vi "Pulse Train demo.vi"() -> ()   [LabVIEW 2019]
doc: "This example shows how to use the Pulse Train VI to construct a series of pulses according to the user-specified pulse prototype."
uses:
  <vilib>/Analysis/1siggen.llb/General Gauss-Mod Sine.vi
  <vilib>/Analysis/1siggen.llb/General Gaussian Monopulse.vi
  <vilib>/Analysis/1siggen.llb/General Aperiodic Triangle.vi
  <vilib>/Analysis/NI_AALBase.lvlib
panel:
  in  "Amplitude & Delay":cluster{"Amplitude":dbl, "Delay (s)":dbl}[](array[cluster])=[{"Amplitude"=5.0, "Delay (s)"=1.0}, {"Amplitude"=3.0, "Delay (s)"=8.0}, {"Amplitude"=1.0, "Delay (s)"=15.0}]
  in  "Stop":bool
  in  "pulse prototype":u16(ring) items=["Gauss Mod-Sine Pattern", "Gauss Monopulse", "Triangle Pattern", "Sine Pattern"]
  in  "interpolation method":i32(ring)=1 items=["nearest", "linear", "spline", "cubic Hermite"]
  out "Pulse Prototype Graph":waveform(dbl)(graph)
  in  "delta t of pulse train":dbl=0.1
  out "Pulse Train":waveform(dbl)(graph)
  # "Overview: This example shows how to use the Pulse Train VI to construct a series of pulses.\nRequirements: LabVIEW Full Development System\nInstructions: \n1.  Run the VI.\n2. Change the pulse parameters, including the pulse prototype, and view the changes in the two graphs.  \n3. Click Stop to stop the VI."
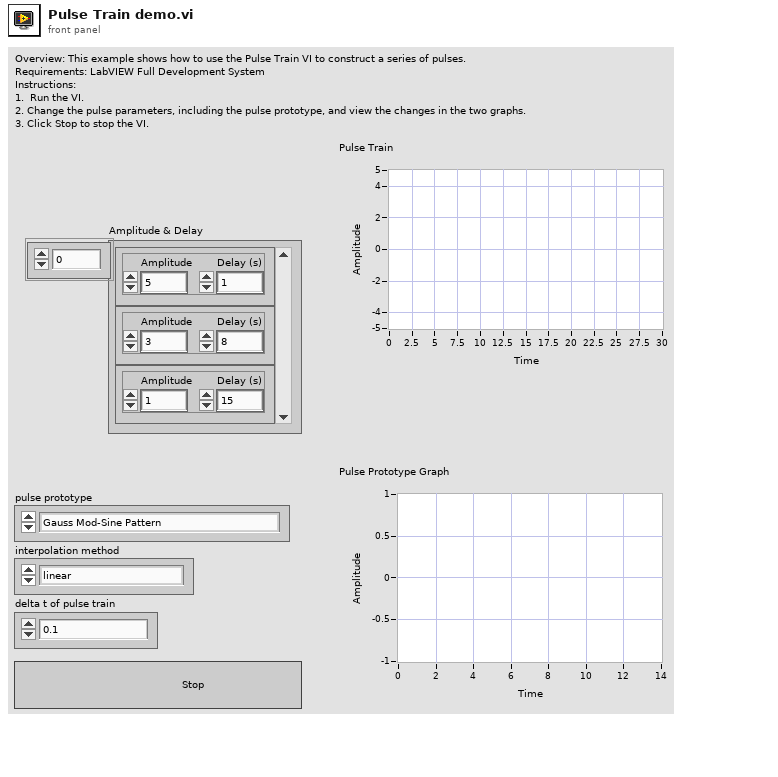
[diagram p1: front panel]
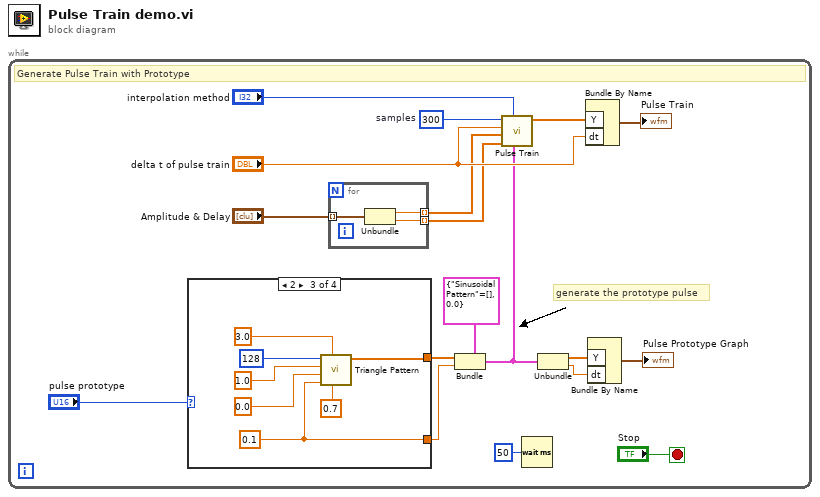
[diagram p0: block diagram]
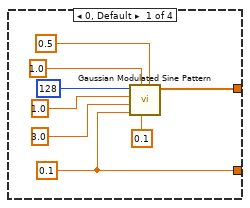
[diagram p2: hidden frame]
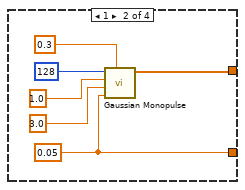
[diagram p3: hidden frame]
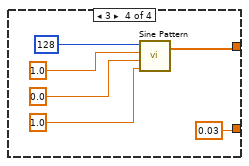
[diagram p4: hidden frame]
diagram:
  n1 = while {
    stop <- "Stop" stop-if-true
    w17 = 300  # samples
    # "generate the prototype pulse"
    # "Generate Pulse Train with Prototype"
    n2 = case shown="2" "pulse prototype" {
      tunnel: [w29 w35 w39 w44] -> w8
      tunnel: [w25 w30 w38 0.03] -> w7
      frame 0, Default {
        w25 = 0.1
        n3 = call <vilib>:"Gaussian Modulated Sine Pattern.vi"("attenuation (dB)"=0.5 ("attenuation"), "normalized bandwidth"=0.1 ("bandwidth"), "center frequency (Hz)"=1.0 ("center frequency"), "delta t (s)"=w25, "delay (s)"=3.0 ("delay"), "amplitude"=1.0, "samples"=128) -> ("Gauss-Mod Sine Pattern"=w29:dbl[])  [unwired: 3 in, 1 out]
      }
      frame 1 {
        w30 = 0.05 ("delta t")
        n4 = call <vilib>:"Gaussian Monopulse.vi"("center frequency (Hz)"=0.3 ("center frequency"), "delta t (s)"=w30, "delay (s)"=3.0 ("delay"), "amplitude"=1.0, "samples"=128) -> ("Gaussian Monopulse"=w35:dbl[])  [unwired: 5 in, 1 out]
      }
      frame 2 {
        w38 = 0.1 ("delta t")
        n5 = call <vilib>:"Triangle Pattern.vi"("asymmetry"=0.7, "width (s)"=3.0 ("width"), "delta t (s)"=w38, "delay (s)"=0.0 ("delay"), "amplitude"=1.0, "samples"=128) -> ("Triangle Pattern"=w39:dbl[])  [unwired: 4 in, 1 out]
      }
      frame 3 {
        n6 = call <vilib>:"Sine Pattern.vi"("cycles"=1.0, "phase(degrees)"=0.0, "amplitude"=1.0, "samples"=128 ("samples 2")) -> ("Sinusoidal Pattern"=w44:dbl[])  [unwired: 1 out]
      }
    }
    n7 = for {
      tunnel: "Amplitude & Delay" -> [w21] mode=indexing
      tunnel: [w20] -> w2 mode=indexing
      tunnel: [w19] -> w1 mode=indexing
      n8 = Unbundle(w21) -> ("Amplitude"=w20:dbl, "Delay (s)"=w19:dbl)
    }
    n9 = Bundle(cluster=cluster{"Sinusoidal Pattern":dbl[], dbl} {"Sinusoidal Pattern"=[], 0.0} ("output cluster"), "Sinusoidal Pattern"=w8, w7) -> (w6:cluster{"Sinusoidal Pattern":dbl[], dbl})
    n10 = call <vilib>:"Pulse Train.vi"("prototype spec"=w6, "interpolation method"="interpolation method", "Delay (s)"=w1, "Amplitude"=w2, "delta t of pulse train (s)"="delta t of pulse train", "samples"=w17) -> ("Pulse Train"=w14:dbl[])  [unwired: 4 in, 1 out]
    n11 = Wait (ms)(milliseconds to wait=u32 50) -> ()  [unwired: 1 out]
    n12 = Unbundle(w6) -> ("Sinusoidal Pattern"=w16:dbl[], w15:dbl)
    n13 = Bundle By Name("Y"=w14, "dt"="delta t of pulse train") -> (→"Pulse Train":waveform(dbl))  [unwired: 1 in]
    n14 = Bundle By Name("Y"=w16, "dt"=w15) -> (→"Pulse Prototype Graph":waveform(dbl))  [unwired: 1 in]
  }
